vi "build output string.vi"(1 "Array of \"period-units\"":i32[](array[numeric])) -> (0 "output string":string)   [LabVIEW 2017]
doc: "Takes an input array x of \"period units\" and builds and output string accordingly. The output string has:\nx(0) number of 0s, then\nx(1) number of 1s, then\nx(2) number of 0s, then\nx(3) number of 1s, and so on."
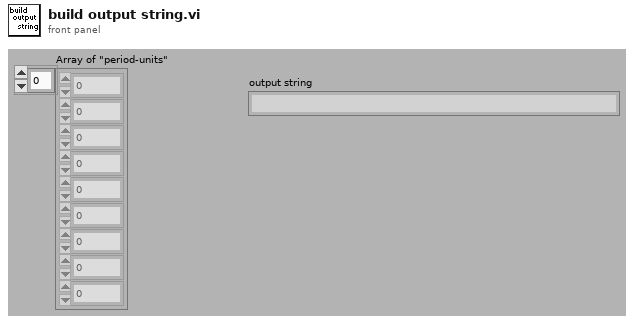
[diagram p1: front panel]
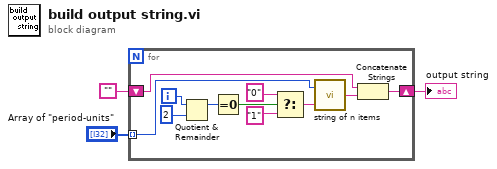
[diagram p0: block diagram]
diagram:
  n1 = for {
    tunnel: "Array of \"period-units\"" -> [w7] mode=indexing
    shift-right: [w5] -> w1
    shift-left: "" -> [w6]
    i -> [w11]
    n2 = Quotient & Remainder(x=w11, y=i8 2) -> (x-y*floor(x/y)=w13:i32)  [unwired: 1 out]
    n3 = Equal To 0?(x=w13) -> (x = 0?=w12:bool)
    n4 = Select(t="0", s=w12, f="1") -> (s? t:f=w10:string)
    n5 = call "string of n items.vi"("string"=w10, "Numeric"=w7) -> ("String"=w4:string)
    n6 = Concatenate Strings(w6, w4) -> (w5:string)
  }
  "output string" <- w1
